vi "Localized Strings.vi"() -> ()   [LabVIEW 2020, in "Message Maker.lvlib"]
uses:
  Message Maker.lvlib
panel:
  in  "Send Overlay":string="Send Overlay"
  in  "Border":string="Border"
  in  "Abstract Message Layer":string="Abstract Message Layer"
  in  "MESSAGES FOR THIS ACTOR":string="MESSAGES FOR THIS ACTOR"
  in  "ABSTRACT MESSAGES FOR CALLER":string="ABSTRACT MESSAGES FOR CALLER"
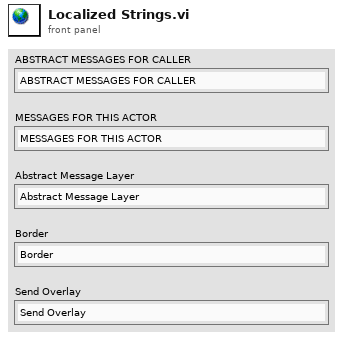
[diagram p1: front panel]
diagram:
